vi "daemon.vi"(8 "error in (no error)":errorcluster, 11 "comic_crawler.lvclass":refnum<class "comic_crawler.lvclass">) -> ()   [LabVIEW 2024, in "comic_crawler.lvclass"]
uses:
  comic_crawler.lvclass
  status--cluster.ctl
  daemon.states--enum.ctl
  comic_crawler.lvclass/comic_crawler.ctl
panel:
  out "status":T1
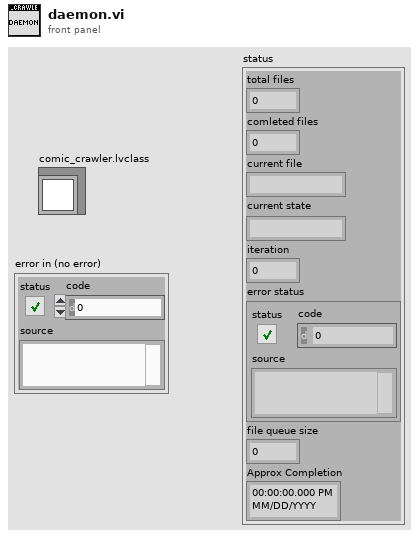
[diagram p1: front panel]
types:
  T1 = typedef "comic_crawler.lvclass/status--cluster.ctl" = cluster{"total files":i32, "comleted files":i32, "current file":string, "current state":string, "iteration":i32, "error status":errorcluster, "file queue size":i32, "Approx Completion":timestamp}
  T2 = typedef "comic_crawler.lvclass/daemon.states--enum.ctl" = enum16{"start search", "idle", "set timer", "running", "stop search", "wait", "set delay", "shut down"}
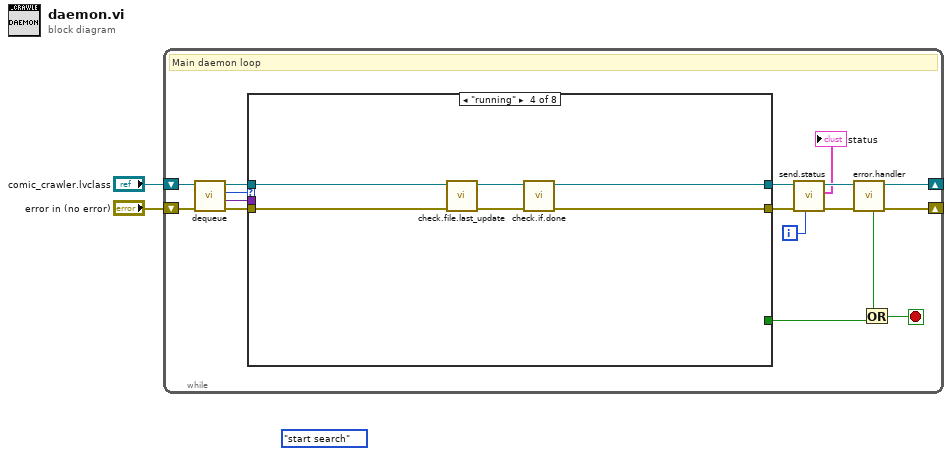
[diagram p0: block diagram]
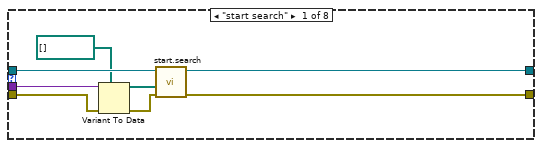
[diagram p2: hidden frame]
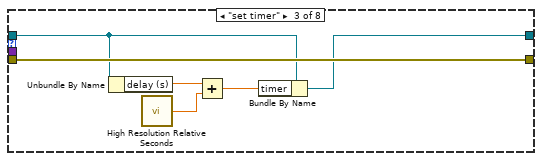
[diagram p4: hidden frame]
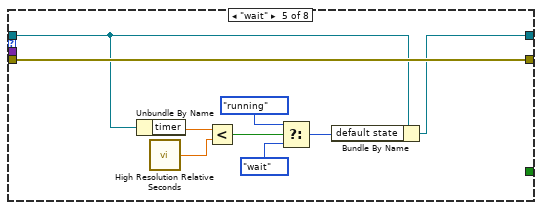
[diagram p5: hidden frame]
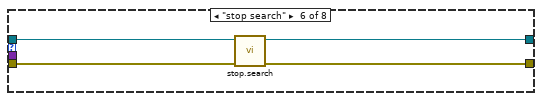
[diagram p6: hidden frame]
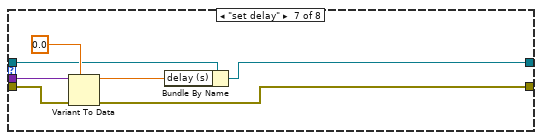
[diagram p7: hidden frame]
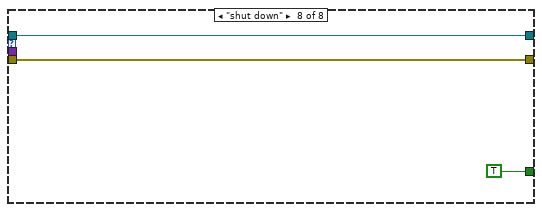
[diagram p8: hidden frame]
diagram:
  (unwired) daemon.states--enum."start search" ("cmd")
  n1 = while {
    shift-right: [w13] -> _
    shift-left: "comic_crawler.lvclass" -> [w19]
    shift-right: [w12] -> _
    shift-left: "error in (no error)" -> [w18]
    i -> [w3]
    stop <- w11 stop-if-true
    # "Main daemon loop"
    n2 = call "dequeue.vi"("error in (no error)"=w18, "comic_crawler.lvclass"=w19) -> ("error out"=w16:errorcluster, "data"=w15:variant, "cmd"=w17:T2, "comic_crawler.lvclass out"=w14:refnum<class "comic_crawler.lvclass">)  [unwired: 6 in]
    n3 = case shown="\"running\"" w17 {
      tunnel: w16 -> [w22 w28 w35 w40 w45 w53 w60 w62]
      tunnel: w15 -> [w24 _ _ _ _ _ w61 _]
      tunnel: w14 -> [w27 w29 w32 w41 w44 w54 w57 w63]
      tunnel: [_ _ _ _ _ _ _ TRUE] -> w10
      tunnel: [w25 w29 w31 w36 w43 w52 w55 w63] -> w8
      tunnel: [w26 w28 w35 w37 w45 w51 w59 w62] -> w6
      frame "start search" {
        n4 = Variant To Data(error in=w22, type=path[] [], Variant=w24) -> (data=w20:path[], error out=w21:errorcluster)
        n5 = call "start.search.vi"("error in (no error)"=w21, "search dirs"=w20, "comic_crawler in"=w27) -> ("error out"=w26:errorcluster, "comic_crawler out"=w25:refnum<class "comic_crawler.lvclass">)  [unwired: 7 in]
      }
      frame "idle" {
      }
      frame "set timer" {
        n6 = Unbundle By Name(w32) -> ("delay (s)"=w34:dbl)
        n7 = call <vilib>:"High Resolution Relative Seconds.vi"() -> ("relative seconds"=w33:dbl)
        n8 = Add(x=w34, y=w33) -> (x+y=w30:dbl)
        n9 = Bundle By Name(cluster=w32, "timer"=w30) -> (w31:refnum<class "comic_crawler.lvclass">)
      }
      frame "running" {
        n10 = call "check.file.last_update.vi"("error in (no error)"=w40, "comic_crawler in"=w41) -> ("error out"=w38:errorcluster, "comic_crawler out"=w39:refnum<class "comic_crawler.lvclass">)  [unwired: 8 in]
        n11 = call "check.if.done.vi"("error in (no error)"=w38, "comic_crawler in"=w39) -> ("error out"=w37:errorcluster, "comic_crawler out"=w36:refnum<class "comic_crawler.lvclass">)  [unwired: 8 in]
      }
      frame "wait" {
        n12 = Unbundle By Name(w44) -> ("timer"=w50:dbl)
        n13 = call <vilib>:"High Resolution Relative Seconds.vi"() -> ("relative seconds"=w49:dbl)
        n14 = Less?(x=w50, y=w49) -> (x < y?=w48:bool)
        n15 = Select(t=daemon.states--enum."running" ("cmd"), s=w48, f=daemon.states--enum."wait" ("cmd")) -> (s? t:f=w42:T2)
        n16 = Bundle By Name(cluster=w44, "default state"=w42) -> (w43:refnum<class "comic_crawler.lvclass">)
      }
      frame "stop search" {
        n17 = call "stop.search.vi"("error in (no error)"=w53, "comic_crawler in"=w54) -> ("error out"=w51:errorcluster, "comic_crawler out"=w52:refnum<class "comic_crawler.lvclass">)  [unwired: 8 in]
      }
      frame "set delay" {
        n18 = Variant To Data(error in=w60, type=0.0, Variant=w61) -> (data=w56:dbl, error out=w59:errorcluster)
        n19 = Bundle By Name(cluster=w57, "delay (s)"=w56) -> (w55:refnum<class "comic_crawler.lvclass">)
      }
      frame "shut down" {
      }
    }
    n20 = call "send.status.vi"("iteration"=w3, "error in (no error)"=w6, "comic_crawler in"=w8) -> ("error out"=w5:errorcluster, "status"=→"status":T1, "comic_crawler out"=w7:refnum<class "comic_crawler.lvclass">)  [unwired: 6 in]
    n21 = call "error.handler.vi"("error in (no error)"=w5, "comic_crawler in"=w7) -> ("error out"=w12:errorcluster, "comic_crawler out"=w13:refnum<class "comic_crawler.lvclass">, "critical"=w9:bool)  [unwired: 7 in]
    n22 = Or(x=w9, y=w10) -> (x .or. y?=w11:bool)
  }
